vi "Saccade suppression - moving grating.vi"() -> ()   [LabVIEW 2013]
uses:
  <vilib>/Platform/TimedLoop/XDataNode/timing_clust.ctl
  <vilib>/Platform/TimedLoop/XDataNode/nitl_modes.ctl
  <vilib>/Platform/TimedLoop/XDataNode/wakeup.ctl
  <vilib>/gmath/statdist.llb/Uniform (Discrete) Random.vi
  Eye tracking dependencies/Global 1.vi
  <vilib>/platform/TimedLoop/XDataNode/XDataNode.xnode
  <vilib>/gmath/NI_Gmath.lvlib
  <vilib>/Platform/TimedLoop/XDataNode/XDNodeRunTimeDep.lvlib
panel:
  in  "Spatial Frequency":sgl=3.0
  in  "Temporal frequency":sgl=3.0
  in  "Contrast":sgl=3.0
  in  "0":bool=TRUE
  in  "1":bool=TRUE
  in  "2":bool=TRUE
  in  "3":bool=TRUE
  in  "4":bool=TRUE
  in  "5":bool=TRUE
  in  "6":bool=TRUE
  in  "7":bool=TRUE
  out "File name exists!":bool
  in  "File name":string="animal15-29_exp1"
  in  "Location":string="D:\\Satoru\\Documents\\Attention_Beh_Data\\"
  out "Std name":string="70915_animal15-21_exp1"
  in  "Save data":bool
  out "State busy":bool
  out "VS busy":bool
  out "LED":bool
  out "State Missed":bool
  out "VS missed":bool
  out "Current trial #":u16
  out "Eye tracker":bool=TRUE
  out "Total number of trials":i32=200
  out "Blank":bool
  in  "Abort":bool caption="run-stop"
  in  "Tab Control":T1(tab)=enum."Network"
  in  "Notes":string
  in  "Start recording @":string
  in  "Inserted probe @":string
  in  "Brain region":string
  in  "Anesthesia @":string
  in  "Anesthesia":string
  in  "Probe configuration":string
  in  "Probe use number":string
  in  "Probe ID":string
  in  "Probe type":string
  in  "Electrode spacing":string
  in  "Electrode area":string
  in  "Penetration angle (to pia)":string
  in  "Penetration coordinates":string
  in  "Penetration distance":string
  in  "Penetration number":string
  in  "Genotype":string
  in  "Transfection":string
  in  "Mass":string
  in  "Sex":string
  in  "Age":string
  in  "Animal ID":string="14-4"
  in  "inter flash interval (ms)":dbl=250.0
  in  "Max jitter (ms)":dbl=250.0
  in  "VS type":string="saccade_grating"
  in  "Background luminance":sgl=60.0
  in  "Pulse amp 0":sgl
  in  "Pulse amp 1":sgl
  in  "Pulse delay (ms)":sgl
  in  "Pulse width (ms)":sgl
  in  "Pulse period":sgl
  in  "Pulse #":sgl
  in  "LED mode":u16(ring) items=["No LED", "Regular", "Random"]
  in  "Chance (%)":dbl
  in  "# of trials":i32=250
  in  "run-stop":bool
  in  "movement":sgl=3.0
  in  "Flash luminance":sgl=190.0
  in  "flash duration (ms)":dbl=16.0
  in  "VS subtype":string="moving"
  in  "Include blanks":bool=TRUE
  in  "# of blank trials":i32=50
  out "Array":bool[](array[boolean])
  in  "Give reward":bool
  in  "Manually give shock":bool
  in  "Water duration (ms)":u32=30
  in  "Shock duration (ms)":u32=10
  in  "Water refractory period (ms)":u32=500
  in  "Shock refractory period (ms)":u32=1000
  in  "Trial timeout (ms)":u32=3000
  in  "Track eye":bool=TRUE
  in  "Allow shock":bool
  in  "Allow timeout":bool
  in  "Manually give water":bool
  in  "Reward period (ms)":u32
  in  "Reward start delay (ms)":u32
  in  "Lick threshold (V)":fxp<+,32,16>=1.600006103515625
  in  "VS threshold (V)":fxp<+,32,16>=0.5
  out "Originating IP":string="192.168.137.2"
  out "Incoming data":string="TrlDone 1.000 "
  in  "Update cycle (ms)":dbl=50.0
  in  "Local IP_This computer":string="192.168.137.10"
  in  "Remote IP_Broadcast":string="192.168.137.255"
  in  "Remote IP_State machine":string="192.168.137.2"
  in  "Remote IP_Visual stimulation":string="192.168.137.3"
  in  "Local port":u16=9090
  in  "Remote port":u16=9091
  out "Error 2":string
  out "Running!":bool
  # "System Status"
  # "VS"
  # "State machine"
  # "Busy"
  # "Missed trial"
  # "Max 20 characters"
  # "(w/o LED)"
  # "Movement threshold (degrees)"
  # "MAX 199.9988"
  # "(This will add trials to the # of trials specified above)"
  # "Errors for debugging"
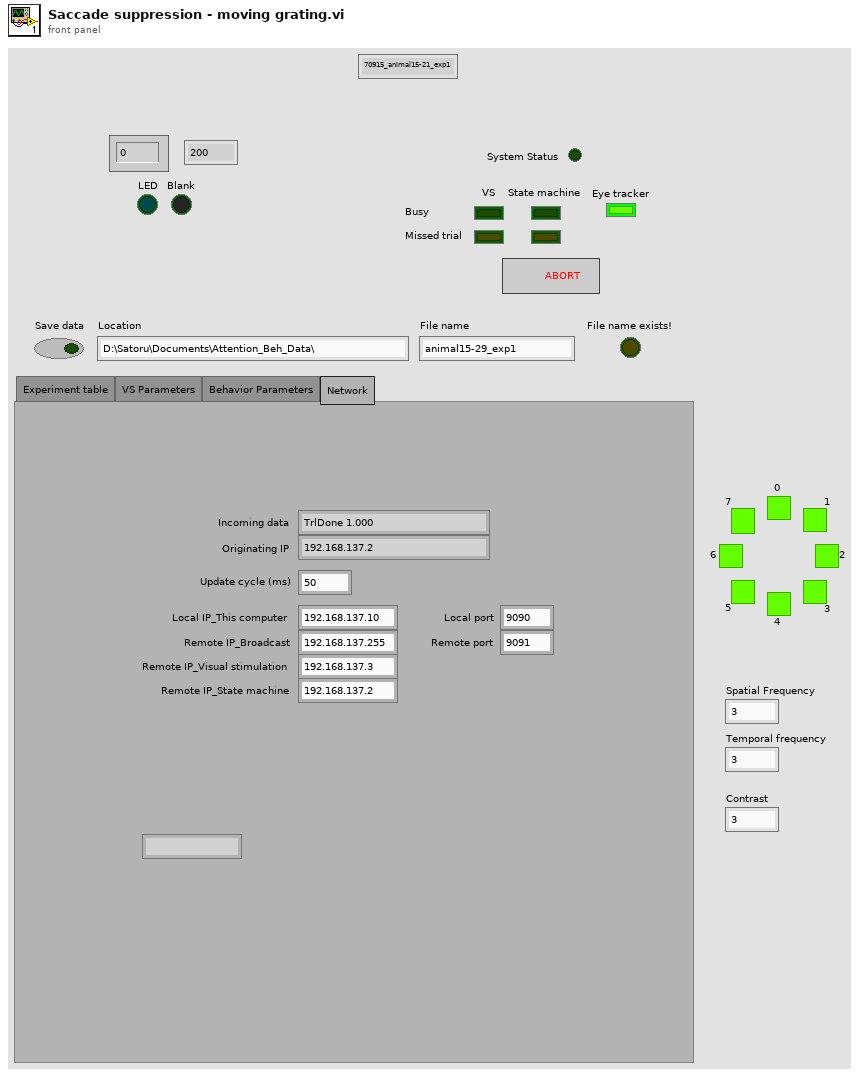
[diagram p1: front panel]
types:
  T1 = enum32{"Experiment table", "VS Parameters", "Behavior Parameters", "Network"}
  T2 = typedef "XDNodeRunTimeDep.lvlib/timing_clust.ctl" = cluster{"Expected End [f-1]":u64, "Actual End [f-1]":u64, "Finished Late? [f-1]":bool, "Expected End [i-1]":u64, "Actual End [i-1]":u64, "Finished Late? [i-1]":bool, "Expected Start [i]":u64, "Actual Start [i]":u64, "Expected Start [f]":u64, "Actual Start [f]":u64, "Source Name":string, "Structure Name":string, "Period":i64, "Deadline":i64, "Offset":i64, "Start":i64, "Priority":i32, "Timeout":i32, "Mode":T3, "Wakeup Reason":T4, "Error":errorcluster, "Source Type":string, "Secondary Source Type":string, "Global End Time":u64, "Global Start Time":u64, "Frame Duration":u64, "Iteration Duration":u64, "Assigned CPU":i32, "I/O Scan Engine Mode":u32}
  T3 = typedef "XDNodeRunTimeDep.lvlib/nitl_modes.ctl" = enum32{"No Change", "Process missed periods, maintain original phase", "Discard missed periods, maintain original phase", "Process missed periods, ignore original phase", "Discard missed periods, ignore original phase"}
  T4 = typedef "XDNodeRunTimeDep.lvlib/wakeup.ctl" = enum32{"Normal", "Aborted", "Asynchronous wakeup", "Timing source error", "Timed loop error", "Timeout"}
  T5 = enum16{"big-endian, network order", "native, host order", "little-endian"}
  T6 = enum16{"open", "replace", "create", "open or create", "replace or create", "replace or create with confirmation"}
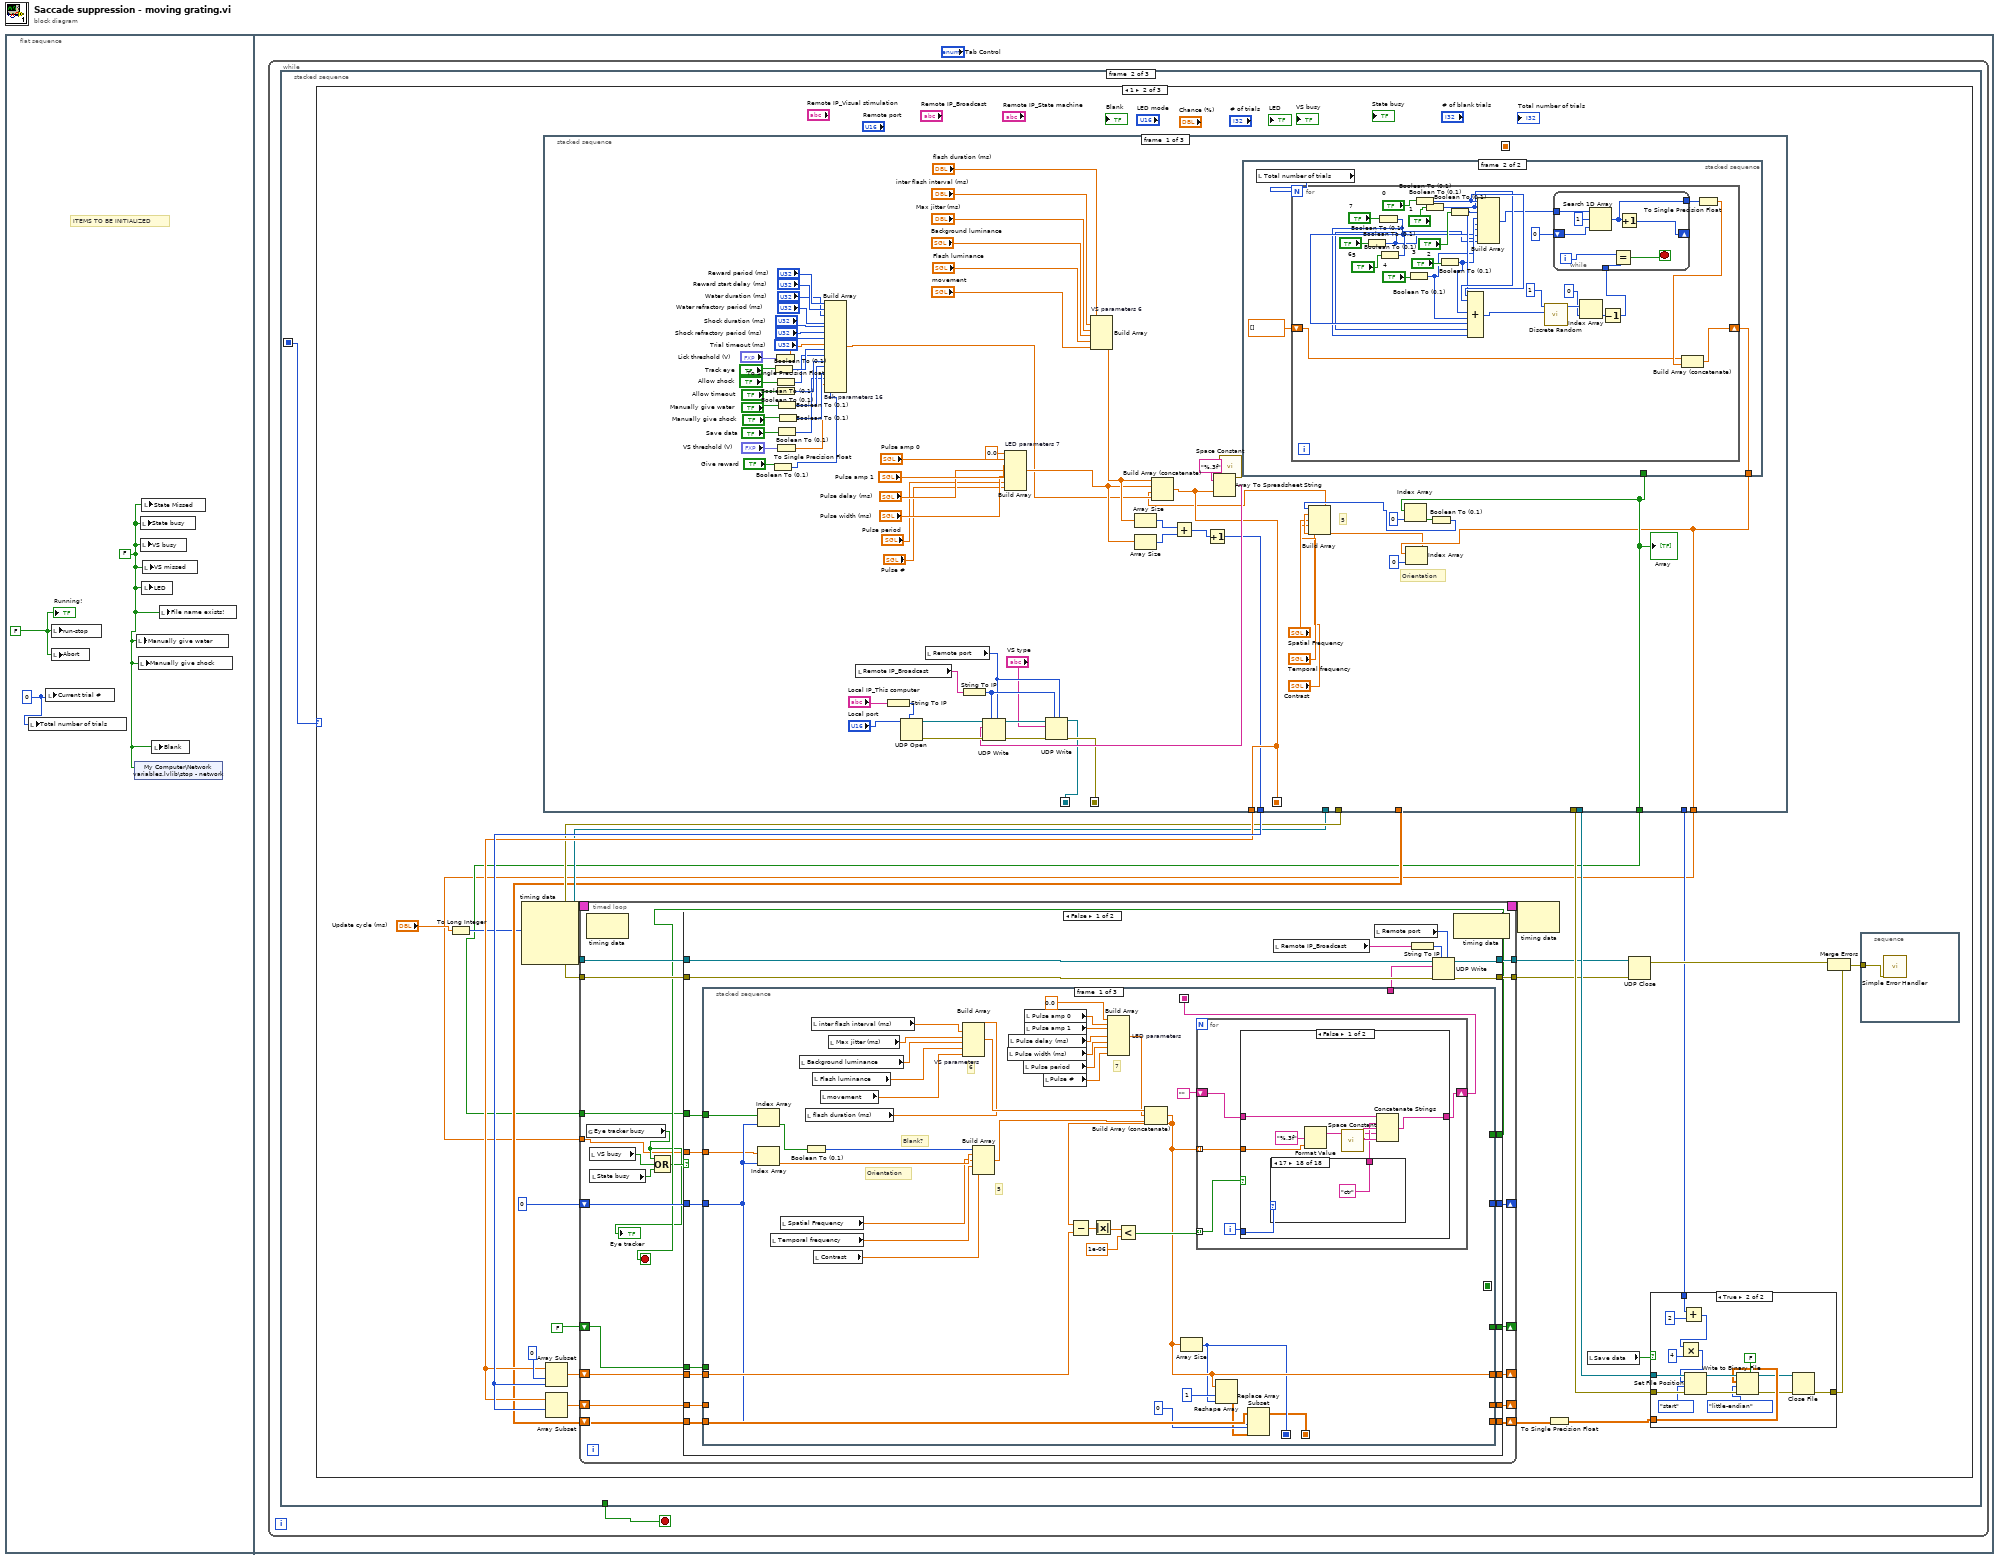
[diagram p0: block diagram]
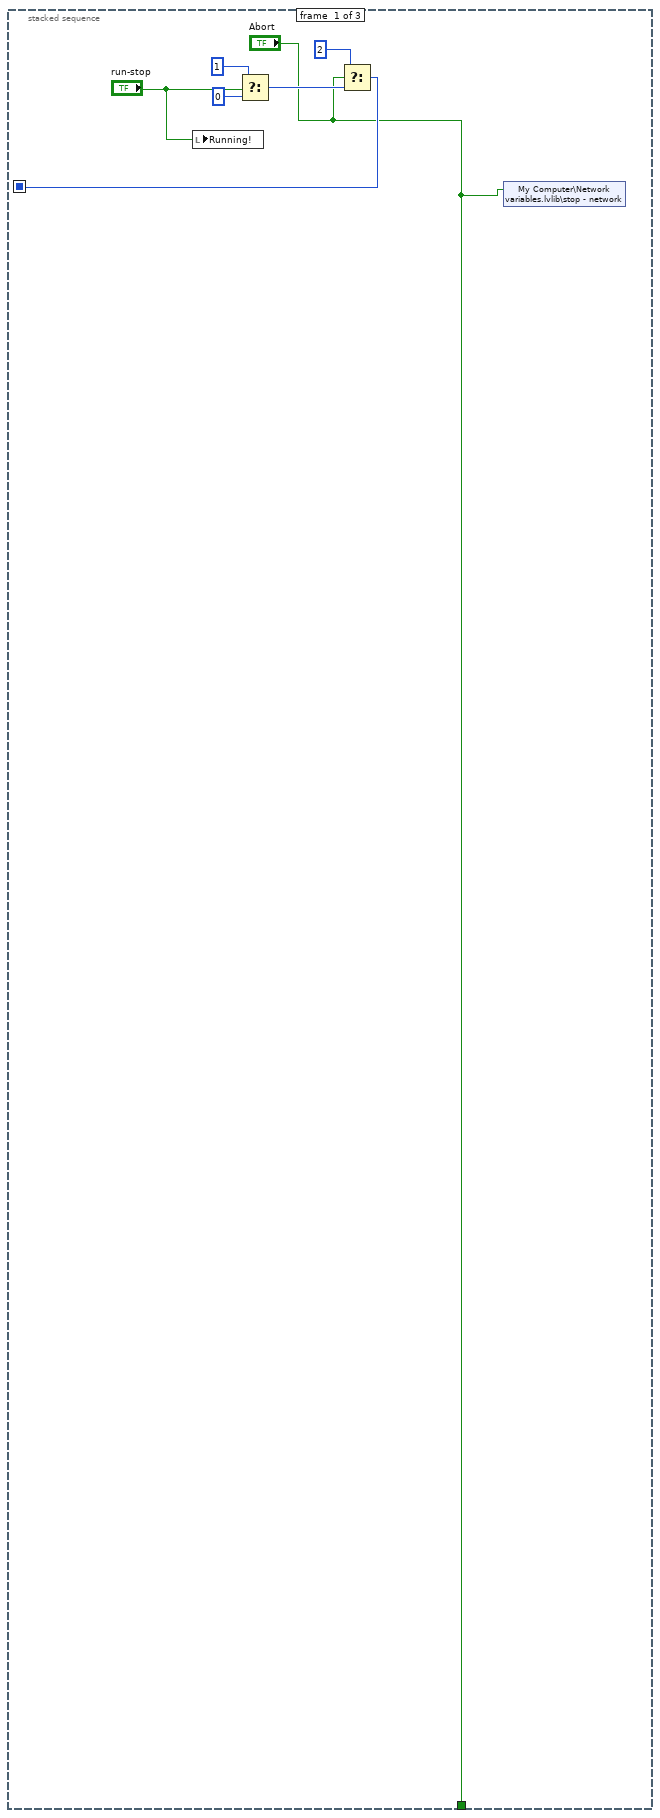
[diagram p2: hidden frame]
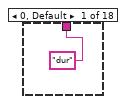
[diagram p4: hidden frame]
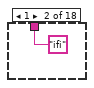
[diagram p5: hidden frame]
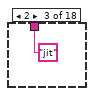
[diagram p6: hidden frame]
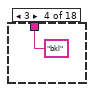
[diagram p7: hidden frame]
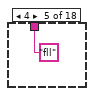
[diagram p8: hidden frame]
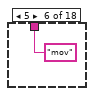
[diagram p9: hidden frame]
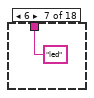
[diagram p10: hidden frame]
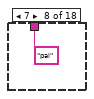
[diagram p11: hidden frame]
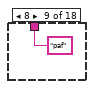
[diagram p12: hidden frame]
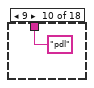
[diagram p13: hidden frame]
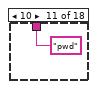
[diagram p14: hidden frame]
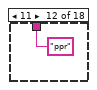
[diagram p15: hidden frame]
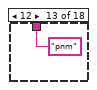
[diagram p16: hidden frame]
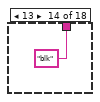
[diagram p17: hidden frame]
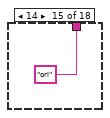
[diagram p18: hidden frame]
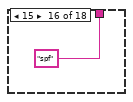
[diagram p19: hidden frame]
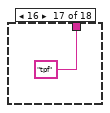
[diagram p20: hidden frame]
diagram:
  n1 = flat-sequence {
    frame #0 {
      w2 = u16 0
      w1 = FALSE ("L dist ind")
      w3 = FALSE
      # "ITEMS TO BE INITIALIZED"
      n2 = local write "Total number of trials"(w2) -> ()
      n3 = local write "Current trial #"(w2) -> ()
      n4 = local write "run-stop"(w3) -> ()
      n5 = local write "Abort"(w3) -> ()
      n6 = shared-variable "My Computer\\Network variables.lvlib\\stop - network"(w1) -> ()  [unwired: 1 in, 1 out]
      n7 = local write "Manually give water"(w1) -> ()
      n8 = local write "Manually give shock"(w1) -> ()
      n9 = local write "State busy"(w1) -> ()
      n10 = local write "VS busy"(w1) -> ()
      n11 = local write "State Missed"(w1) -> ()
      n12 = local write "LED"(w1) -> ()
      n13 = local write "VS missed"(w1) -> ()
      n14 = local write "Blank"(w1) -> ()
      n15 = local write "File name exists!"(w1) -> ()
      "Running!" <- w3
    }
    frame #1 {
      n16 = while {
        stop <- w4 stop-if-true
        n17 = stacked-sequence {
          seq-local: [w7 _ _] -> [_ w12 _]
          tunnel: ["Abort" _ _] -> w4
          frame #0 {
            n18 = local write "Running!"("run-stop") -> ()
            n19 = Select(t=u8 1, s="run-stop", f=u8 0) -> (s? t:f=w8:u8)
            n20 = Select(t=u8 2, s="Abort", f=w8) -> (s? t:f=w7:u8)
            n21 = shared-variable "My Computer\\Network variables.lvlib\\stop - network"("Abort") -> ()  [unwired: 1 in, 1 out]
          }
          frame #1 {
            n22 = case shown="1" w12 {
              frame 0, Default {
              }
              frame 1 {
                n23 = To Long Integer(number="Update cycle (ms)") -> (32bit integer=w22:i32)
                n24 = node-c288(w22) -> (w39:T2)  [unwired: 3 in]
                n25 = stacked-sequence {
                  seq-local: [w449 _ _] -> [_ _ w629]
                  seq-local: [_ w571 _] -> [_ _ w620]
                  seq-local: [w461 _ _] -> [_ _ w618]
                  seq-local: [w460 _ _] -> [_ _ w604]
                  tunnel: [w449 _ _] -> w34
                  tunnel: [w446 _ _] -> w35
                  tunnel: [_ _ w602] -> w31
                  tunnel: [_ _ w601] -> w30
                  tunnel: [_ _ w623] -> w29
                  tunnel: [_ _ w622] -> w25
                  tunnel: [_ _ w621] -> w24
                  tunnel: [_ _ w599] -> w15
                  tunnel: [w450 _ _] -> w14
                  tunnel: [w444 _ _] -> w13
                  frame #0 {
                    # "5"
                    # "Orientation"
                    n26 = Boolean To (0,1)(Boolean="Give reward") -> (0, 1=w462:i16)
                    n27 = Boolean To (0,1)(Boolean="Track eye") -> (0, 1=w502:i16)
                    n28 = To Single Precision Float(number="Lick threshold (V)") -> (single precision float=w467:sgl)
                    n29 = Boolean To (0,1)(Boolean="Allow shock") -> (0, 1=w500:i16)
                    n30 = Boolean To (0,1)(Boolean="Allow timeout") -> (0, 1=w498:i16)
                    n31 = Boolean To (0,1)(Boolean="Manually give water") -> (0, 1=w496:i16)
                    n32 = Boolean To (0,1)(Boolean="Save data") -> (0, 1=w493:i16)
                    n33 = To Single Precision Float(number="VS threshold (V)") -> (single precision float=w464:sgl)
                    n34 = Boolean To (0,1)(Boolean="Manually give shock") -> (0, 1=w495:i16)
                    n35 = Build Array "Beh parameters 16"("Reward period (ms)", "Reward start delay (ms)", "Water duration (ms)", "Water refractory period (ms)", "Shock duration (ms)", "Shock refractory period (ms)", "Trial timeout (ms)", w467, w502, w500, w498, w496, w495, w493, w464, w462) -> (w448:sgl[])
                    n36 = local read "Remote IP_Broadcast"() -> (w480:string)
                    n37 = String To IP(1:"Local IP_This computer") -> (0:w484:u32)
                    n38 = UDP Open(7:w484, 11:"Local port") -> (port=w481:refnum<k16>, 0:w485:errorcluster)  [unwired: 3 in, 1 out]
                    n39 = local read "Remote port"() -> (w475:u16)
                    n40 = String To IP(1:w480) -> (0:w476:u32)
                    n41 = Build Array "LED parameters 7"(sgl 0.0 ("element"), "Pulse amp 0", "Pulse amp 1", "Pulse delay (ms)", "Pulse width (ms)", "Pulse period", "Pulse #") -> (w470:sgl[])
                    n42 = Build Array "VS parameters 6"("flash duration (ms)", "inter flash interval (ms)", "Max jitter (ms)", "Background luminance", "Flash luminance", "movement") -> (w471:dbl[])
                    n43 = Array Size(array=w471) -> (size(s)=w469:i32)
                    n44 = Array Size(array=w470) -> (size(s)=w468:i32)
                    n45 = Add(x=w469, y=w468) -> (x+y=w447:i32)
                    n46 = Increment(x=w447) -> (x+1=w446:i32)
                    n47 = call <vilib>:"Space Constant.vi"() -> ("String"=w478:string)
                    n48 = stacked-sequence {
                      tunnel: [w511 _] -> w450
                      tunnel: [_ w531] -> w444
                      frame #0 {
                        n49 = case shown="True" "Include blanks" {
                          tunnel: [w513 w517] -> w511
                          frame False {
                            n50 = local read "# of trials"() -> (w515:i32)
                            n51 = Initialize Array(FALSE, w515) -> (w513:bool[])
                            n52 = local write "Total number of trials"(w515) -> ()
                          }
                          frame True {
                            n53 = local read "# of blank trials"() -> (w519:i32)
                            n54 = local read "# of trials"() -> (w516:i32)
                            n55 = Add(x=w516, y=w519) -> (x+y=w518:i32)
                            n56 = local write "Total number of trials"(w518) -> ()
                            n57 = Initialize Array(FALSE, w516) -> (w520:bool[])
                            n58 = for {
                              N: w519 -> [_]
                              shift-right: [w524] -> w517
                              shift-left: w520 -> [w525]
                              n59 = Array Size(array=w525) -> (size(s)=w529:i32)
                              n60 = call-poly <vilib>:"Discrete Random.vi"("n"=w529, "samples"=1) -> ("uniform (discrete) random data"=w528:i32[])  [unwired: 8 in, 1 out]
                              n61 = Index Array(array=w528, index=0) -> (element=w526:i32)
                              n62 = Decrement(x=w526) -> (x-1=w523:i32)
                              n63 = Insert Into Array(array=w525, index=w523, new element=TRUE) -> (w524:bool[])
                            }
                          }
                        }
                      }
                      frame #1 {
                        n64 = local read "Total number of trials"() -> (w533:i32)
                        n65 = for {
                          N: w533 -> [_]
                          shift-right: [w534] -> w531
                          shift-left: sgl[] [] ("array type (2D Dbl)") -> [w535]
                          n66 = Boolean To (0,1)(Boolean="6") -> (0, 1=w543:i16)
                          n67 = Boolean To (0,1)(Boolean="7") -> (0, 1=w542:i16)
                          n68 = Boolean To (0,1)(Boolean="5") -> (0, 1=w544:i16)
                          n69 = Boolean To (0,1)(Boolean="4") -> (0, 1=w545:i16)
                          n70 = Boolean To (0,1)(Boolean="0") -> (0, 1=w549:i16)
                          n71 = Boolean To (0,1)(Boolean="1") -> (0, 1=w548:i16)
                          n72 = Boolean To (0,1)(Boolean="3") -> (0, 1=w546:i16)
                          n73 = Boolean To (0,1)(Boolean="2") -> (0, 1=w547:i16)
                          n74 = Compound Arithmetic op=ADD(w549, w548, w547, w546, w545, w544, w543, w542) -> (w541:i16)
                          n75 = Build Array(w549, w548, w547, w546, w545, w544, w543, w542) -> (w540:i16[])
                          n76 = call-poly <vilib>:"Discrete Random.vi"("n"=w541, "samples"=1) -> ("uniform (discrete) random data"=w560:i32[])  [unwired: 8 in, 1 out]
                          n77 = Index Array(array=w560, index=0) -> (element=w558:i32)
                          n78 = Decrement(x=w558) -> (x-1=w539:i32)
                          n79 = while {
                            tunnel: w540 -> [w569]
                            tunnel: [w567] -> w537
                            tunnel: w539 -> [w565]
                            shift-right: [w562] -> _
                            shift-left: 0 -> [w563]
                            i -> [w566]
                            stop <- w564 stop-if-true
                            n80 = Search 1D Array(1D array=w569, element=i16 1, start index (0)=w563) -> (index of element=w567:i32)
                            n81 = Equal?(x=w566, y=w565) -> (x = y?=w564:bool)
                            n82 = Increment(x=w567) -> (x+1=w562:i32)
                          }
                          n83 = To Single Precision Float(number=w537) -> (single precision float=w536:sgl)
                          n84 = Build Array (concatenate)(w535, w536) -> (w534:sgl[])
                        }
                      }
                    }
                    "Array" <- w450
                    n85 = Index Array(array=w450, index=0) -> (element=w451:bool)
                    n86 = Index Array(array=w444, index=0) -> (element=w442:sgl)
                    n87 = Boolean To (0,1)(Boolean=w451) -> (0, 1=w443:i16)
                    n88 = Build Array(w443, w442, "Spatial Frequency", "Temporal frequency", "Contrast") -> (w441:sgl[])
                    n89 = Build Array (concatenate)(w471, w470, w441, w448) -> (w449:dbl[])
                    n90 = Array To Spreadsheet String(delimiter (Tab)=w478, array=w449, 3:"%.3f" ("format string")) -> (spreadsheet string=w477:string)
                    n91 = UDP Write(address=w476, port or service name=w475, connection ID=w481, data in=w477, 8:w485) -> (error out=w474:errorcluster, 3:w473:refnum<k16>)  [unwired: 1 in]
                    n92 = UDP Write(address=w476, port or service name=w475, connection ID=w473, data in="VS type", 8:w474) -> (error out=w461:errorcluster, 3:w460:refnum<k16>)  [unwired: 1 in]
                  }
                  frame #1 {
                    w578 = "&" ("string")
                    # "state definition"
                    n93 = local read "inter flash interval (ms)"() -> (w593:dbl)
                    n94 = local read "Total number of trials"() -> (w570:i32)
                    n95 = local read "Max jitter (ms)"() -> (w592:dbl)
                    n96 = local read "VS subtype"() -> (w597:string)
                    n97 = local read "Chance (%)"() -> (w591:dbl)
                    n98 = local read "LED mode"() -> (w594:u16)
                    n99 = local read "VS type"() -> (w598:string)
                    n100 = String To Byte Array(string=w598) -> (unsigned byte array=w596:u8[])
                    n101 = String To Byte Array(string=w597) -> (unsigned byte array=w595:u8[])
                    n102 = Concatenate Strings("idle", w578, "vs before", w578, "vs", w578, "vs after", w578, "cycle end", w578, "reward", w578, "reward refractory", w578, "punish", w578, "punish refractory", w578, "exit", w578, "timeout", w578) -> (w579:string)
                    n103 = Build Array (concatenate)(w596, w595, w594, w570, w593, w592, w591) -> (w575:dbl[])
                    n104 = String To Byte Array(string=w579) -> (unsigned byte array=w573:u8[])
                    n105 = Initialize Array(sgl 0.0 ("element"), 37 ("dimension size")) -> (w574:sgl[])
                    n106 = Build Array (concatenate)(w575, w574, w573) -> (w572:dbl[])
                    n107 = To Single Precision Float(number=w572) -> (single precision float=w571:sgl[])
                  }
                  frame #2 {
                    # "# of parameters, column"
                    n108 = local read "Save data"() -> (w626:bool)
                    n109 = local read "Remote IP_Broadcast"() -> (w612:string)
                    n110 = local read "Remote port"() -> (w610:u16)
                    n111 = String To IP(1:w612) -> (0:w611:u32)
                    n112 = local read "Total number of trials"() -> (w619:i32)
                    n113 = Array Size(array=w629) -> (size(s)=w627:i32)
                    n114 = Build Array(w619, w627) -> (w625:i32[])
                    n115 = Initialize Array(sgl 0.0, w619, w627) -> (w623:sgl[][])
                    n116 = To Single Precision Float(number=w625) -> (single precision float=w624:sgl[])
                    n117 = case shown="True" w626 {
                      tunnel: w624 -> [_ w702]
                      tunnel: w623 -> [_ w701]
                      tunnel: [_ w700] -> w622
                      tunnel: [_ w699] -> w621
                      tunnel: w620 -> [_ w698]
                      tunnel: ["" w634] -> w606
                      tunnel: [_ w633] -> w599
                      frame False {
                      }
                      frame True {
                        w669 = 20 ("dimension size")
                        w639 = 500 ("dimension size")
                        w641 = T5."little-endian" ("byte order (0:big-endian, network order)")
                        w711 = enum16{"start", "end", "current"}."start" ("from (0:start)")
                        # "param array"
                        # "row and col\nfor param array"
                        # "first 500 singles for common params"
                        # "reserve 500 singles"
                        # "write behhavior params"
                        # "datapath"
                        n118 = while {
                          tunnel: [w742] -> w704
                          tunnel: [w741] -> w703
                          tunnel: [w734] -> w634
                          stop <- w739 continue-if-true
                          (unwired) "0" ("replace string (\"\")")
                          w763 = "/"
                          n119 = Get Date/Time String() -> (date string=w765:string)  [unwired: 3 in, 1 out]
                          n120 = Match Pattern(string=w765, regular expression=w763) -> (before substring=w762:string, after substring=w764:string)  [unwired: 1 in, 2 out]
                          n121 = Decimal String To Number(string=w762) -> (number=w757:i32)  [unwired: 2 in, 1 out]
                          n122 = Match Pattern(string=w764, regular expression=w763) -> (before substring=w761:string, after substring=w751:string)  [unwired: 1 in, 2 out]
                          n123 = Number To Decimal String(number=w757, width (-)=i16 2) -> (decimal integer string=w759:string)
                          n124 = call <vilib>:"Space Constant.vi"() -> ("String"=w758:string)
                          n125 = Decimal String To Number(string=w761) -> (number=w754:i32)  [unwired: 2 in, 1 out]
                          n126 = Search and Replace String(input string=w759, search string=w758) -> (result string=w749:string)  [unwired: 6 in, 3 out]
                          n127 = Number To Decimal String(number=w754, width (-)=i16 2) -> (decimal integer string=w756:string)
                          n128 = String Subset(string=w751, offset (0)=2) -> (substring=w747:string)  [unwired: 1 in]
                          n129 = call <vilib>:"Space Constant.vi"() -> ("String"=w755:string)
                          n130 = Search and Replace String(input string=w756, search string=w755, replace string="0" ("replace string (\"\")")) -> (result string=w748:string)  [unwired: 5 in, 3 out]
                          n131 = Concatenate Strings(w749, w748, w747) -> (w737:string)
                          n132 = Concatenate Strings(w737, "_" ("string"), "File name") -> (w734:string)
                          "Std name" <- w734
                          n133 = Concatenate Strings("Location", w737, "_" ("string"), "File name", ".beh" ("string")) -> (w744:string)
                          n134 = Wait (ms)(milliseconds to wait=u32 100) -> ()  [unwired: 1 out]
                          n135 = String To Path(string=w744) -> (path=w743:path)
                          n136 = call <vilib>:"Check if File or Folder Exists.vi"("path"=w743) -> ("error out"=w741:errorcluster, "file or folder exists?"=w739:bool, "dup path"=w742:path)  [unwired: 8 in]
                          "File name exists!" <- w739
                        }
                        n137 = String To Byte Array(string="Animal ID") -> (unsigned byte array=w661:u8[])
                        n138 = String To Byte Array(string="Genotype") -> (unsigned byte array=w652:u8[])
                        n139 = String To Byte Array(string="Age") -> (unsigned byte array=w653:u8[])
                        n140 = String To Byte Array(string="Sex") -> (unsigned byte array=w654:u8[])
                        n141 = String To Byte Array(string="Mass") -> (unsigned byte array=w655:u8[])
                        n142 = String To Byte Array(string="Transfection") -> (unsigned byte array=w656:u8[])
                        n143 = String To Byte Array(string="Penetration number") -> (unsigned byte array=w658:u8[])
                        n144 = String To Byte Array(string="Penetration distance") -> (unsigned byte array=w660:u8[])
                        n145 = String To Byte Array(string="Penetration coordinates") -> (unsigned byte array=w684:u8[])
                        n146 = String To Byte Array(string="Penetration angle (to pia)") -> (unsigned byte array=w685:u8[])
                        n147 = String To Byte Array(string="Electrode area") -> (unsigned byte array=w686:u8[])
                        n148 = String To Byte Array(string="Electrode spacing") -> (unsigned byte array=w687:u8[])
                        n149 = String To Byte Array(string="Probe type") -> (unsigned byte array=w688:u8[])
                        n150 = String To Byte Array(string="Probe ID") -> (unsigned byte array=w689:u8[])
                        n151 = String To Byte Array(string="Probe use number") -> (unsigned byte array=w690:u8[])
                        n152 = String To Byte Array(string="Probe configuration") -> (unsigned byte array=w691:u8[])
                        n153 = String To Byte Array(string="Anesthesia") -> (unsigned byte array=w692:u8[])
                        n154 = String To Byte Array(string="Anesthesia @") -> (unsigned byte array=w693:u8[])
                        n155 = String To Byte Array(string="Brain region") -> (unsigned byte array=w694:u8[])
                        n156 = String To Byte Array(string="Inserted probe @") -> (unsigned byte array=w695:u8[])
                        n157 = String To Byte Array(string="Start recording @") -> (unsigned byte array=w696:u8[])
                        n158 = String To Byte Array(string="Notes") -> (unsigned byte array=w697:u8[])
                        n159 = Build Array(w661, w652, w653, w654, w655, w656, w658, w660, w684, w685, w686, w687, w688, w689, w690, w691, w692, w693, w694, w695, w696, w697) -> (w664:u8[][])
                        n160 = for {
                          tunnel: w664 -> [w731] mode=indexing
                          tunnel: [w730] -> w662 mode=indexing
                          tunnel: w669 -> [w729]
                          n161 = Initialize Array(u8 0 ("element"), w729) -> (w733:u8[])
                          n162 = Replace Array Subset(array=w733, new element=w731) -> (w730:u8[])  [unwired: 1 in]
                        }
                        n163 = Array Size(array=w664) -> (size(s)=w666:i32[])
                        n164 = Index Array(array=w666, index=0) -> (element=w668:i32)
                        n165 = Open/Create/Replace File(file path (use dialog)=w704, error in=w703, operation (0:open)=T6."create", access (0:read/write)=enum16{"read/write", "read-only", "write-only"}."write-only") -> (refnum out=w725:refnum<file>, error out=w724:errorcluster)  [unwired: 2 in, 1 out]
                        n166 = Multiply(x=w669, y=w668) -> (x*y=w637:i32)
                        n167 = Set File Position(offset (in bytes) (0)=i64 0, refnum=w725, from (0:start)=w711, error in=w724) -> (refnum out=w645:refnum<file>, error out=w643:errorcluster)
                        n168 = To Single Precision Float(number=w662) -> (single precision float=w663:sgl[][])
                        n169 = Initialize Array(sgl 0.0 ("element"), w639) -> (w721:sgl[])
                        n170 = Reshape Array(w663, 1 ("dimension size"), w637) -> (w640:sgl[][])
                        n171 = Write to Binary File(file (use dialog)=w645, data=w640, error in=w643, 5:FALSE ("prepend array or string size? (T)"), 9:w641) -> (refnum out=w644:refnum<file>, error out=w642:errorcluster)  [unwired: 1 in, 1 out]
                        n172 = Write to Binary File(file (use dialog)=w644, data=w721, error in=w642, 5:FALSE ("prepend array or string size? (T)"), 9:w641) -> (refnum out=w719:refnum<file>, error out=w718:errorcluster)  [unwired: 1 in, 1 out]
                        n173 = Multiply(x=w637, y=4) -> (x*y=w638:i32)
                        n174 = Set File Position(offset (in bytes) (0)=w638, refnum=w719, from (0:start)=w711, error in=w718) -> (refnum out=w717:refnum<file>, error out=w716:errorcluster)
                        n175 = Add(x=w637, y=w639) -> (x+y=w633:i32)
                        n176 = Write to Binary File(file (use dialog)=w717, data=w698, error in=w716, 5:FALSE ("prepend array or string size? (T)"), 9:w641) -> (refnum out=w715:refnum<file>, error out=w714:errorcluster)  [unwired: 1 in, 1 out]
                        n177 = Multiply(x=w633, y=4) -> (x*y=w713:i32)
                        n178 = Set File Position(offset (in bytes) (0)=w713, refnum=w715, from (0:start)=w711, error in=w714) -> (refnum out=w709:refnum<file>, error out=w708:errorcluster)
                        n179 = Write to Binary File(file (use dialog)=w709, data=w702, error in=w708, 5:FALSE ("prepend array or string size? (T)"), 9:w641) -> (refnum out=w707:refnum<file>, error out=w706:errorcluster)  [unwired: 1 in, 1 out]
                        n180 = Write to Binary File(file (use dialog)=w707, data=w701, error in=w706, 5:FALSE ("prepend array or string size? (T)"), 9:w641) -> (refnum out=w699:refnum<file>, error out=w700:errorcluster)  [unwired: 1 in, 1 out]
                      }
                    }
                    n181 = String Length(string=w606) -> (length=w609:i32)
                    n182 = Not Equal To 0?(x=w609) -> (x != 0?=w608:bool)
                    n183 = Select(t=w606, s=w608, f="Test") -> (s? t:f=w605:string)
                    n184 = UDP Write(address=w611, port or service name=w610, connection ID=w604, data in=w605, 8:w618) -> (error out=w617:errorcluster, 3:w603:refnum<k16>)  [unwired: 1 in]
                    n185 = UDP Write(address=w611, port or service name=w610, connection ID=w603, data in="VS subtype", 8:w617) -> (error out=w613:errorcluster, 3:w601:refnum<k16>)  [unwired: 1 in]
                    n186 = Unbundle By Name(w613) -> ("code"=w616:i32)
                    n187 = Equal?(x=w616, y=56) -> (x = y?=w614:bool)
                    n188 = case shown="True" w614 {
                      tunnel: w613 -> [w630 _]
                      tunnel: [w630 errorcluster {"status"=FALSE, "code"=0, "source"=""} ("error out")] -> w602
                      frame False {
                      }
                      frame True {
                      }
                    }
                  }
                }
                n189 = Array Subset(array=w34, index=0, length=w35) -> (w37:dbl[])
                n190 = Array Subset(array=w34, index=w35) -> (w33:dbl[])  [unwired: 1 in]
                n191 = timed-loop {
                  shift-right: [w59] -> _
                  shift-left: u16 0 -> [w58]
                  tunnel: w31 -> [w57]
                  tunnel: w30 -> [w56]
                  tunnel: [w55] -> w16
                  tunnel: [w54] -> w17
                  shift-right: [w53] -> _
                  shift-left: w37 -> [w61]
                  shift-right: [w52] -> _
                  shift-left: w33 -> [w60]
                  shift-right: [w50] -> w28
                  shift-left: w29 -> [w51]
                  shift-right: [w49] -> _
                  shift-left: FALSE -> [w48]
                  timing: w39 -> [_]
                  timing-out: [_] -> w38
                  tunnel: w14 -> [w42]
                  tunnel: w13 -> [w41]
                  stop <- w47 stop-if-true
                  n192 = node-c288() -> ()  [unwired: 1 in, 1 out]
                  n193 = global read "Global 1.vi" "Eye tracker busy"() -> (w43:bool)
                  "Eye tracker" <- w43
                  n194 = local read "VS busy"() -> (w45:bool)
                  n195 = local read "State busy"() -> (w44:bool)
                  n196 = Compound Arithmetic op=OR(w43, w45, w44) -> (w46:bool)
                  n197 = case shown="False" w46 {
                    tunnel: w61 -> [w84 w270]
                    tunnel: w60 -> [w83 w268]
                    tunnel: [w82 w259] -> w59
                    tunnel: w58 -> [w81 w260]
                    tunnel: w57 -> [w77 w266]
                    tunnel: w56 -> [w76 w264]
                    tunnel: [w75 w265] -> w55
                    tunnel: [w74 w263] -> w54
                    tunnel: [w73 w270] -> w53
                    tunnel: [w72 w261] -> w52
                    tunnel: w51 -> [w71 w269]
                    tunnel: [w70 w269] -> w50
                    tunnel: [w69 w262] -> w49
                    tunnel: w48 -> [w68 w267]
                    tunnel: [w66 FALSE] -> w47
                    tunnel: w42 -> [w65 _]
                    tunnel: w41 -> [w64 _]
                    frame False {
                      n198 = stacked-sequence {
                        seq-local: [w110 _ _] -> [_ w181 _]
                        seq-local: [w103 _ _] -> [_ w175 _]
                        seq-local: [w102 _ _] -> [_ w174 _]
                        seq-local: [_ w164 _] -> [_ _ w251]
                        tunnel: w81 -> [w92 w162 w253]
                        tunnel: w84 -> [w115 _ _]
                        tunnel: w83 -> [_ w188 _]
                        tunnel: [_ _ w252] -> w82
                        tunnel: [w107 _ _] -> w73
                        tunnel: [_ w171 _] -> w72
                        tunnel: w71 -> [w106 _ _]
                        tunnel: [_ w169 _] -> w70
                        tunnel: [_ w164 _] -> w69
                        tunnel: w68 -> [_ w165 _]
                        tunnel: [_ w163 _] -> w67
                        tunnel: [_ w156 _] -> w66
                        tunnel: w65 -> [w94 _ _]
                        tunnel: w64 -> [w91 _ _]
                        frame #0 {
                          # "5"
                          # "Blank?"
                          # "Orientation"
                          # "6"
                          # "7"
                          n199 = Index Array(array=w94, index=w92) -> (element=w93:bool)
                          n200 = Index Array(array=w91, index=w92) -> (element=w88:sgl)
                          n201 = local read "Temporal frequency"() -> (w86:sgl)
                          n202 = local read "Spatial Frequency"() -> (w87:sgl)
                          n203 = local read "Background luminance"() -> (w99:sgl)
                          n204 = Boolean To (0,1)(Boolean=w93) -> (0, 1=w89:i16)
                          n205 = local read "flash duration (ms)"() -> (w95:dbl)
                          n206 = local read "inter flash interval (ms)"() -> (w101:dbl)
                          n207 = local read "Flash luminance"() -> (w98:sgl)
                          n208 = local read "Contrast"() -> (w85:sgl)
                          n209 = local read "movement"() -> (w97:sgl)
                          n210 = local read "Max jitter (ms)"() -> (w100:dbl)
                          n211 = Build Array "VS parameters"(w95, w101, w100, w99, w98, w97) -> (w117:dbl[])
                          n212 = Build Array(w89, w88, w87, w86, w85) -> (w90:sgl[])
                          n213 = local read "Pulse width (ms)"() -> (w121:sgl)
                          n214 = local read "Pulse delay (ms)"() -> (w120:sgl)
                          n215 = local read "Pulse period"() -> (w122:sgl)
                          n216 = local read "Pulse amp 0"() -> (w118:sgl)
                          n217 = local read "Pulse amp 1"() -> (w119:sgl)
                          n218 = local read "Pulse #"() -> (w123:sgl)
                          n219 = Build Array "LED parameters"(sgl 0.0 ("element"), w118, w119, w120, w121, w122, w123) -> (w116:sgl[])
                          n220 = Build Array (concatenate)(w117, w116, w90) -> (w107:dbl[])
                          n221 = Subtract(x=w107, y=w115) -> (x-y=w114:dbl[])
                          n222 = Absolute Value(x=w114) -> (abs(x)=w112:dbl[])
                          n223 = Less?(x=w112, y=1e-06) -> (x < y?=w111:bool[])
                          n224 = Array Size(array=w107) -> (size(s)=w103:i32)
                          n225 = for {
                            tunnel: w111 -> [w128] mode=indexing
                            shift-right: [w126] -> w110
                            shift-left: "" -> [w127]
                            tunnel: w107 -> [w125] mode=indexing
                            i -> [w124]
                            n226 = case shown="False" w128 {
                              tunnel: w127 -> [w136 w155]
                              tunnel: [w135 w155] -> w126
                              tunnel: w124 -> [w133 _]
                              tunnel: w125 -> [w129 _]
                              frame False {
                                n227 = case shown="17" w133 {
                                tunnel: ["dur" "ifi" "jit" "bkl" "fll" "mov" "led" "pai" "paf" "pdl" "pwd" "ppr" "pnm" "blk" "ori" "spf" "tpf" "ctr"] -> w132
                                frame 0, Default {
                                }
                                frame 1 {
                                }
                                frame 2 {
                                }
                                frame 3 {
                                }
                                frame 4 {
                                }
                                frame 5 {
                                }
                                frame 6 {
                                }
                                frame 7 {
                                }
                                frame 8 {
                                }
                                frame 9 {
                                }
                                frame 10 {
                                }
                                frame 11 {
                                }
                                frame 12 {
                                }
                                frame 13 {
                                }
                                frame 14 {
                                }
                                frame 15 {
                                }
                                frame 16 {
                                }
                                frame 17 {
                                }
                                }
                                n228 = Format Value(format string="%.3f", value (0)=w129) -> (output string=w130:string)  [unwired: 1 in]
                                n229 = call <vilib>:"Space Constant.vi"() -> ("String"=w134:string)
                                n230 = Concatenate Strings(w136, w132, w134, w130, w134) -> (w135:string)
                              }
                              frame True {
                              }
                            }
                          }
                          n231 = Reshape Array(w107, 1 ("dimension size"), w103) -> (w104:dbl[][])
                          n232 = Replace Array Subset(array=w106, new element=w104, index (row)=w92, index (col)=0) -> (w102:sgl[][])
                        }
                        frame #1 {
                          # "16"
                          n233 = local read "Manually give shock"() -> (w192:bool)
                          n234 = local read "Manually give water"() -> (w194:bool)
                          n235 = local read "Shock refractory period (ms)"() -> (w202:u32)
                          n236 = local read "Lick threshold (V)"() -> (w182:fxp<+,32,16>)
                          n237 = local read "Water refractory period (ms)"() -> (w204:u32)
                          n238 = local read "VS threshold (V)"() -> (w160:fxp<+,32,16>)
                          n239 = local read "Allow timeout"() -> (w196:bool)
                          n240 = local read "Give reward"() -> (w158:bool)
                          n241 = local read "Reward start delay (ms)"() -> (w206:u32)
                          n242 = local read "Allow shock"() -> (w198:bool)
                          n243 = local read "Save data"() -> (w190:bool)
                          n244 = local read "Shock duration (ms)"() -> (w203:u32)
                          n245 = local read "Track eye"() -> (w199:bool)
                          n246 = local read "Water duration (ms)"() -> (w205:u32)
                          n247 = local read "Reward period (ms)"() -> (w207:u32)
                          n248 = local read "Trial timeout (ms)"() -> (w201:u32)
                          n249 = Boolean To (0,1)(Boolean=w158) -> (0, 1=w157:i16)
                          n250 = Boolean To (0,1)(Boolean=w199) -> (0, 1=w200:i16)
                          n251 = Boolean To (0,1)(Boolean=w198) -> (0, 1=w197:i16)
                          n252 = Boolean To (0,1)(Boolean=w196) -> (0, 1=w195:i16)
                          n253 = Boolean To (0,1)(Boolean=w194) -> (0, 1=w193:i16)
                          n254 = Boolean To (0,1)(Boolean=w192) -> (0, 1=w191:i16)
                          n255 = Boolean To (0,1)(Boolean=w190) -> (0, 1=w189:i16)
                          n256 = To Single Precision Float(number=w182) -> (single precision float=w183:sgl)
                          n257 = To Single Precision Float(number=w160) -> (single precision float=w159:sgl)
                          n258 = Build Array "Beh parameters"(w207, w206, w205, w204, w203, w202, w201, w183, w200, w197, w195, w193, w191, w189, w159, w157) -> (w171:sgl[])
                          n259 = Subtract(x=w171, y=w188) -> (x-y=w187:dbl[])
                          n260 = Array Size(array=w171) -> (size(s)=w172:i32)
                          n261 = Absolute Value(x=w187) -> (abs(x)=w185:dbl[])
                          n262 = Less?(x=w185, y=1e-06) -> (x < y?=w184:bool[])
                          n263 = Reshape Array(w171, 1 ("dimension size"), w172) -> (w170:sgl[][])
                          n264 = local read "Total number of trials"() -> (w161:i32)
                          n265 = for {
                            tunnel: w184 -> [w224] mode=indexing
                            tunnel: w171 -> [w223] mode=indexing
                            shift-right: [w221] -> w180
                            shift-left: w181 -> [w222]
                            i -> [w225]
                            n266 = case shown="False" w224 {
                              tunnel: w225 -> [w233 _]
                              tunnel: w223 -> [w231 _]
                              tunnel: w222 -> [w228 w250]
                              tunnel: [w226 w250] -> w221
                              frame False {
                                n267 = case shown="0, Default" w233 {
                                tunnel: ["rwp" "rwd" "wdr" "wre" "shd" "shr" "tto" "lkt" "etk" "ash" "ato" "gwt" "gsh" "sav" "vsh" "rew"] -> w227
                                frame 0, Default {
                                }
                                frame 1 {
                                }
                                frame 2 {
                                }
                                frame 3 {
                                }
                                frame 4 {
                                }
                                frame 5 {
                                }
                                frame 6 {
                                }
                                frame 7 {
                                }
                                frame 8 {
                                }
                                frame 9 {
                                }
                                frame 10 {
                                }
                                frame 11 {
                                }
                                frame 12 {
                                }
                                frame 13 {
                                }
                                frame 14 {
                                }
                                frame 15 {
                                }
                                }
                                n268 = Format Value(format string="%.3f", value (0)=w231) -> (output string=w229:string)  [unwired: 1 in]
                                n269 = call <vilib>:"Space Constant.vi"() -> ("String"=w230:string)
                                n270 = Concatenate Strings(w228, w227, w230, w229, w230) -> (w226:string)
                              }
                              frame True {
                              }
                            }
                          }
                          n271 = local read "Current trial #"() -> (w176:u16)
                          n272 = local read "run-stop"() -> (w168:bool)
                          n273 = local read "State Missed"() -> (w178:bool)
                          n274 = local read "VS missed"() -> (w177:bool)
                          n275 = Not(x=w168) -> (.not. x?=w167:bool)
                          n276 = Equal?(x=w176, y=w161) -> (x = y?=w179:bool)
                          n277 = Compound Arithmetic op=OR(w177, w178, w179) -> (w166:bool)
                          n278 = case shown="True" w166 {
                            frame False {
                            }
                            frame True {
                              w208 = FALSE
                              n279 = local write "Running!"(w208) -> ()
                              n280 = local write "run-stop"(w208) -> ()
                            }
                          }
                          n281 = Compound Arithmetic op=OR(w166, w167, w165) -> (w164:bool)
                          n282 = case shown="False" w164 {
                            tunnel: w180 -> [w215 _]
                            tunnel: [w211 w217] -> w163
                            tunnel: [FALSE TRUE] -> w156
                            frame False {
                              n283 = call <vilib>:"Space Constant.vi"() -> ("String"=w213:string)
                              n284 = Concatenate Strings(w215, "start", w213, "1.000", w213) -> (w211:string)
                              n285 = global write "Global 1.vi" "Start one trial"(TRUE) -> ()
                            }
                            frame True {
                              n286 = call <vilib>:"Space Constant.vi"() -> ("String"=w219:string)
                              n287 = Concatenate Strings("stop", w219, "1.000", w219) -> (w217:string)
                            }
                          }
                          n288 = Replace Array Subset(array=w174, new element=w170, index (row)=w162, index (col)=w175) -> (w169:sgl[][])
                        }
                        frame #2 {
                          n289 = case shown="False" w251 {
                            tunnel: w253 -> [w256 w257]
                            tunnel: [w255 w257] -> w252
                            frame False {
                              w254 = TRUE
                              n290 = Increment(x=w256) -> (x+1=w255:u16)
                              "Current trial #" <- w255
                              n291 = local write "VS busy"(w254) -> ()
                              n292 = local write "State busy"(w254) -> ()
                            }
                            frame True {
                            }
                          }
                        }
                      }
                      n293 = local read "Remote IP_Broadcast"() -> (w78:string)
                      n294 = local read "Remote port"() -> (w80:u16)
                      n295 = String To IP(1:w78) -> (0:w79:u32)
                      n296 = UDP Write(address=w79, port or service name=w80, connection ID=w76, data in=w67, 8:w77) -> (error out=w75:errorcluster, 3:w74:refnum<k16>)  [unwired: 1 in]
                    }
                    frame True {
                      n297 = stacked-sequence {
                        seq-local: [w278 _] -> [_ w374]
                        seq-local: [w277 _] -> [_ w375]
                        tunnel: w268 -> [w294 _]
                        tunnel: w267 -> [w285 _]
                        tunnel: w266 -> [w284 _]
                        tunnel: [_ w369] -> w265
                        tunnel: w264 -> [w283 _]
                        tunnel: [_ w366] -> w263
                        tunnel: [w271 _] -> w262
                        tunnel: [w279 _] -> w261
                        tunnel: w260 -> [_ w363]
                        tunnel: [_ w361] -> w259
                        frame #0 {
                          n298 = local read "Manually give shock"() -> (w304:bool)
                          n299 = local read "Manually give water"() -> (w306:bool)
                          n300 = local read "Shock refractory period (ms)"() -> (w314:u32)
                          n301 = local read "Lick threshold (V)"() -> (w295:fxp<+,32,16>)
                          n302 = local read "Water refractory period (ms)"() -> (w316:u32)
                          n303 = local read "VS threshold (V)"() -> (w275:fxp<+,32,16>)
                          n304 = local read "Allow timeout"() -> (w308:bool)
                          n305 = local read "Reward start delay (ms)"() -> (w318:u32)
                          n306 = local read "Allow shock"() -> (w310:bool)
                          n307 = local read "Save data"() -> (w302:bool)
                          n308 = local read "Shock duration (ms)"() -> (w315:u32)
                          n309 = local read "Track eye"() -> (w311:bool)
                          n310 = local read "Water duration (ms)"() -> (w317:u32)
                          n311 = local read "Reward period (ms)"() -> (w319:u32)
                          n312 = local read "Trial timeout (ms)"() -> (w313:u32)
                          n313 = Boolean To (0,1)(Boolean=w311) -> (0, 1=w312:i16)
                          n314 = Boolean To (0,1)(Boolean=w310) -> (0, 1=w309:i16)
                          n315 = Boolean To (0,1)(Boolean=w308) -> (0, 1=w307:i16)
                          n316 = Boolean To (0,1)(Boolean=w306) -> (0, 1=w305:i16)
                          n317 = Boolean To (0,1)(Boolean=w304) -> (0, 1=w303:i16)
                          n318 = Boolean To (0,1)(Boolean=w302) -> (0, 1=w301:i16)
                          n319 = To Single Precision Float(number=w295) -> (single precision float=w296:sgl)
                          n320 = To Single Precision Float(number=w275) -> (single precision float=w274:sgl)
                          n321 = local read "Give reward"() -> (w273:bool)
                          n322 = Boolean To (0,1)(Boolean=w273) -> (0, 1=w272:i16)
                          n323 = Build Array "Beh parameters"(w319, w318, w317, w316, w315, w314, w313, w296, w312, w309, w307, w305, w303, w301, w274, w272) -> (w279:sgl[])
                          n324 = Subtract(x=w279, y=w294) -> (x-y=w300:dbl[])
                          n325 = Absolute Value(x=w300) -> (abs(x)=w298:dbl[])
                          n326 = Less?(x=w298, y=1e-06) -> (x < y?=w297:bool[])
                          n327 = for {
                            tunnel: w297 -> [w334] mode=indexing
                            tunnel: w279 -> [w333] mode=indexing
                            shift-right: [w331] -> w280
                            shift-left: "" -> [w332]
                            i -> [w335]
                            n328 = case shown="False" w334 {
                              tunnel: w335 -> [w343 _]
                              tunnel: w333 -> [w341 _]
                              tunnel: w332 -> [w338 w360]
                              tunnel: [w336 w360] -> w331
                              frame False {
                                n329 = case shown="0, Default" w343 {
                                tunnel: ["rwp" "rwd" "wdr" "wre" "shd" "shr" "tto" "lkt" "etk" "ash" "ato" "gwt" "gsh" "sav" "vst" "rew"] -> w337
                                frame 0, Default {
                                }
                                frame 1 {
                                }
                                frame 2 {
                                }
                                frame 3 {
                                }
                                frame 4 {
                                }
                                frame 5 {
                                }
                                frame 6 {
                                }
                                frame 7 {
                                }
                                frame 8 {
                                }
                                frame 9 {
                                }
                                frame 10 {
                                }
                                frame 11 {
                                }
                                frame 12 {
                                }
                                frame 13 {
                                }
                                frame 14 {
                                }
                                frame 15 {
                                }
                                }
                                n330 = Format Value(format string="%.3f", value (0)=w341) -> (output string=w339:string)  [unwired: 1 in]
                                n331 = call <vilib>:"Space Constant.vi"() -> ("String"=w340:string)
                                n332 = Concatenate Strings(w338, w337, w340, w339, w340) -> (w336:string)
                              }
                              frame True {
                              }
                            }
                          }
                          n333 = String Length(string=w280) -> (length=w281:i32)
                          n334 = Not Equal To 0?(x=w281) -> (x != 0?=w282:bool)
                          n335 = case shown="True" w282 {
                            tunnel: w284 -> [w320 w326]
                            tunnel: [w320 w325] -> w277
                            tunnel: w283 -> [w321 w324]
                            tunnel: [w321 w323] -> w278
                            tunnel: w280 -> [_ w322]
                            frame False {
                            }
                            frame True {
                              n336 = local read "Remote IP_Broadcast"() -> (w327:string)
                              n337 = local read "Remote port"() -> (w329:u16)
                              n338 = String To IP(1:w327) -> (0:w328:u32)
                              n339 = UDP Write(address=w328, port or service name=w329, connection ID=w324, data in=w322, 8:w326) -> (error out=w325:errorcluster, 3:w323:refnum<k16>)  [unwired: 1 in]
                            }
                          }
                          n340 = local read "Total number of trials"() -> (w276:i32)
                          n341 = local read "Current trial #"() -> (w289:u16)
                          n342 = local read "run-stop"() -> (w288:bool)
                          n343 = local read "State Missed"() -> (w291:bool)
                          n344 = local read "VS missed"() -> (w290:bool)
                          n345 = Not(x=w288) -> (.not. x?=w287:bool)
                          n346 = Equal?(x=w289, y=w276) -> (x = y?=w292:bool)
                          n347 = Compound Arithmetic op=OR(w290, w291, w292) -> (w286:bool)
                          n348 = Compound Arithmetic op=OR(w286, w287, w285) -> (w271:bool)
                          n349 = case shown="True" w271 {
                            frame False {
                            }
                            frame True {
                              w330 = FALSE
                              n350 = local write "Running!"(w330) -> ()
                              n351 = local write "run-stop"(w330) -> ()
                            }
                          }
                        }
                        frame #1 {
                          n352 = UDP Read(connection ID=w374, timeout ms (25000)=0, 8:w375) -> (data out=w362:string, error out=w370:errorcluster, 3:w366:refnum<k16>, 6:w364:u32)  [unwired: 1 in, 1 out]
                          n353 = Unbundle By Name(w370) -> ("code"=w371:i32)
                          n354 = Equal?(x=w371, y=56) -> (x = y?=w373:bool)
                          n355 = case shown="True" w373 {
                            tunnel: w370 -> [w415 _]
                            tunnel: [w415 errorcluster {"status"=FALSE, "code"=0, "source"=""} ("error out")] -> w369
                            frame False {
                            }
                            frame True {
                            }
                          }
                          n356 = String Length(string=w362) -> (length=w368:i32)
                          n357 = Not Equal To 0?(x=w368) -> (x != 0?=w367:bool)
                          n358 = case shown="True" w367 {
                            tunnel: w364 -> [_ w380]
                            tunnel: w363 -> [w376 w379]
                            tunnel: w362 -> [_ w384]
                            tunnel: [w376 w377] -> w361
                            frame False {
                            }
                            frame True {
                              (unwired) -1.0 ("default value 2")
                              (unwired) "no" ("default value 1")
                              n359 = Scan From String(format string="%s %f ", input string=w384, initial scan location=u32 0) -> (output 1=w381:string, output 2=w378:dbl)  [unwired: 3 in, 3 out]
                              n360 = case shown="\"TrlDone\", Default" w381 {
                                tunnel: w380 -> [w392]
                                tunnel: w379 -> [w385]
                                tunnel: w378 -> [w387]
                                tunnel: [w385] -> w377
                                frame "TrlDone", Default {
                                n361 = local read "Remote IP_State machine"() -> (w389:string)
                                n362 = IP To String(1:TRUE ("dot notation? (F)"), 2:w392) -> (0:w386:string)
                                "Originating IP" <- w386
                                n363 = Match True/False String(2:"" ("false string"), 3:w389, 4:w386) -> (0:w388:bool)  [unwired: 1 out]
                                n364 = case shown="False" w388 {
                                tunnel: w385 -> [w393 w412]
                                tunnel: w387 -> [w394 w413]
                                tunnel: w386 -> [w398 _]
                                frame False {
                                n365 = local read "Remote IP_Visual stimulation"() -> (w396:string)
                                n366 = Match True/False String(2:"" ("false string"), 3:w396, 4:w398) -> (0:w395:bool)  [unwired: 1 out]
                                n367 = case shown="True" w395 {
                                tunnel: w394 -> [_ w403]
                                tunnel: w393 -> [_ w402]
                                frame False {
                                "Error 2" <- "Unknown source Error"
                                }
                                frame True {
                                n368 = Subtract(x=w403, y=w402) -> (x-y=w406:dbl)
                                n369 = global write "Global 1.vi" "camera stop"(TRUE ("dot notation? (F)")) -> ()
                                n370 = Absolute Value(x=w406) -> (abs(x)=w405:dbl)
                                n371 = local write "VS busy"(FALSE) -> ()
                                n372 = Greater?(x=w405, y=1e-06) -> (0:→"VS missed":bool)
                                }
                                }
                                }
                                frame True {
                                n373 = Subtract(x=w413, y=w412) -> (x-y=w411:dbl)
                                n374 = local write "State busy"(FALSE) -> ()
                                n375 = Absolute Value(x=w411) -> (abs(x)=w410:dbl)
                                n376 = Greater?(x=w410, y=1e-06) -> (0:→"State Missed":bool)
                                }
                                }
                                }
                              }
                              "Incoming data" <- w384
                            }
                          }
                        }
                      }
                    }
                  }
                  n377 = node-c288() -> ()  [unwired: 1 in, 1 out]
                }
                n378 = node-c288(w38) -> ()  [unwired: 1 out]
                n379 = To Single Precision Float(number=w28) -> (single precision float=w23:sgl[][])
                n380 = local read "Save data"() -> (w26:bool)
                n381 = UDP Close(connection ID=w17, 8:w16) -> (error out=w21:errorcluster)  [unwired: 1 out]
                n382 = case shown="True" w26 {
                  tunnel: w25 -> [w421 w437]
                  tunnel: w24 -> [_ w436]
                  tunnel: w23 -> [_ w428]
                  tunnel: [w421 w425] -> w20
                  tunnel: w15 -> [_ w424]
                  frame False {
                  }
                  frame True {
                    n383 = Add(x=w424, y=2) -> (x+y=w422:i32)
                    n384 = Multiply(x=w422, y=4) -> (x*y=w433:i32)
                    n385 = Set File Position(offset (in bytes) (0)=w433, refnum=w436, from (0:start)=enum16{"start", "end", "current"}."start", error in=w437) -> (refnum out=w430:refnum<file>, error out=w431:errorcluster)
                    n386 = Write to Binary File(file (use dialog)=w430, data=w428, error in=w431, 5:FALSE ("prepend array or string size? (T)"), 9:T5."little-endian" ("byte order (0:big-endian, network order)")) -> (refnum out=w426:refnum<file>, error out=w427:errorcluster)  [unwired: 1 in, 1 out]
                    n387 = Close File(refnum=w426, error in=w427) -> (error out=w425:errorcluster)  [unwired: 1 out]
                  }
                }
                n388 = Merge Errors(w21, w20) -> (w19:errorcluster)
                n389 = stacked-sequence {
                  tunnel: w19 -> [w40]
                  frame #0 {
                    n390 = call <vilib>:"Simple Error Handler.vi"("error in (no error)"=w40) -> ()  [unwired: 4 in, 5 out]
                  }
                }
              }
              frame 2 {
              }
            }
          }
          frame #2 {
            n391 = Wait (ms)(milliseconds to wait=u32 100) -> ()  [unwired: 1 out]
          }
        }
      }
    }
  }
